vi "subGetItemInfosFromProjectRef.vi"(9 "All Files in Dir":path[](array[path]), 10 "Source dist":map{string, set{string}}(c390), 11 "TargetFile info in":T1) -> (1 "Project refs":refnum<vi>[](array[refnum]), 2 "Local Host App Instance":refnum<vi>, 3 "TargetFile info":T1)   [LabVIEW 2020, in "SolutionBuilder.lvlib"]
uses:
  SolutionBuilder.lvlib
  ItemInfo.ctl
  ProjectInfo.ctl
  FileInfo.ctl
  <vilib>/Utility/miscctls.llb/LVMapReplaceAction.ctl
  2df07852-fbbc-4590-81e1-2119d6acaec0.vi
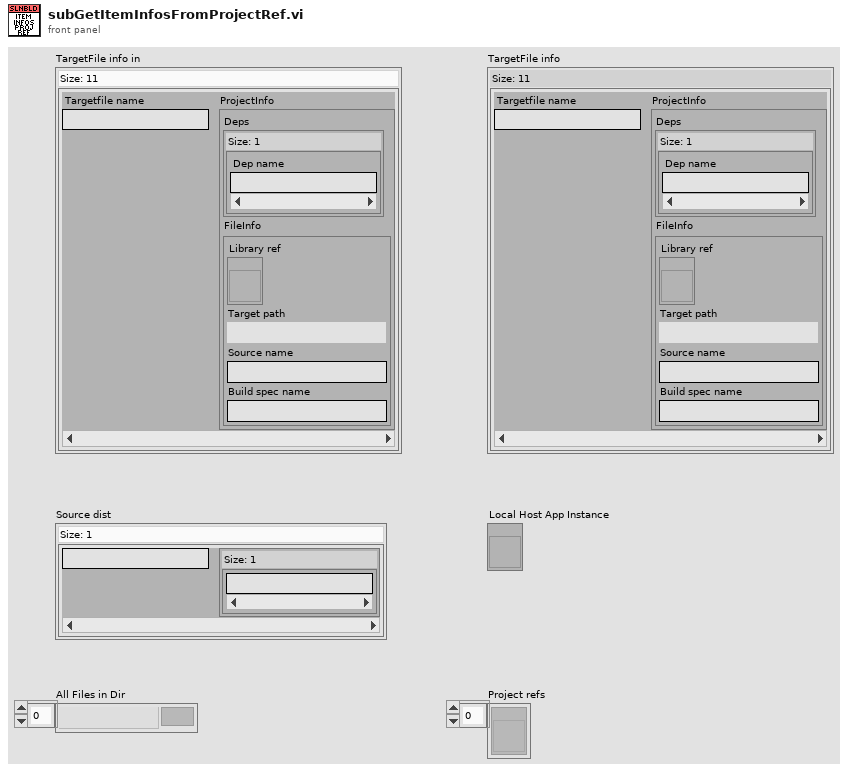
[diagram p1: front panel]
types:
  T1 = typedef "SolutionBuilder.lvlib/ItemInfo.ctl" = map{string, T2}
  T2 = typedef "SolutionBuilder.lvlib/ProjectInfo.ctl" = cluster{"Deps":set{string}, "FileInfo":T3}
  T3 = typedef "SolutionBuilder.lvlib/FileInfo.ctl" = cluster{"Library ref":refnum<vi>, "Target path":path, "Source name":string, "Build spec name":string}
  T4 = typedef "LVMapReplaceAction.ctl" = enum32{"Modify Entry only if found", "Add or Modify Entry", "Delete Entry"}
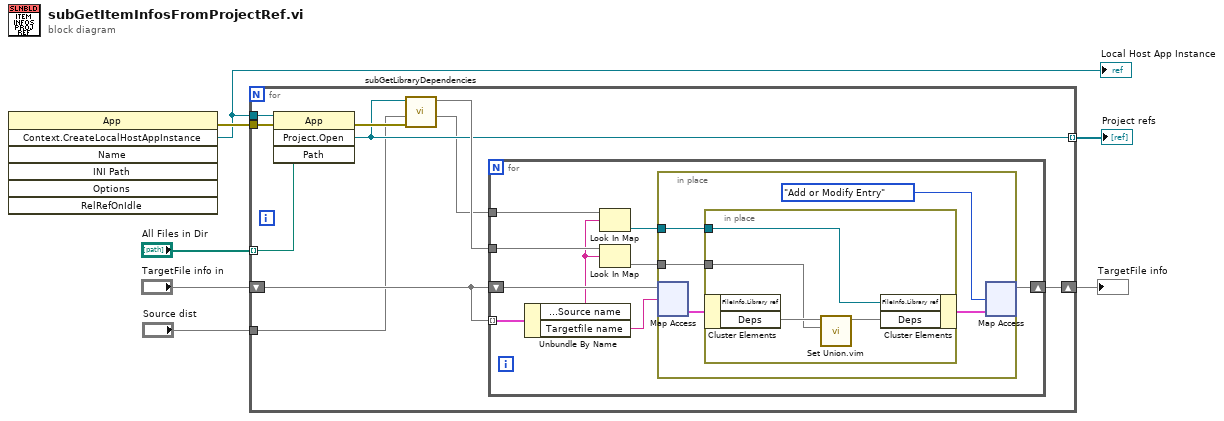
[diagram p0: block diagram]
diagram:
  n1 = invoke class="App" method="Context.CreateLocalHostAppInstance"() -> (error out=w6:errorcluster, "Create Context"=w5:refnum<vi>)  [unwired: 7 in, 5 out]
  "Local Host App Instance" <- w5
  n2 = for {
    tunnel: "All Files in Dir" -> [w17] mode=indexing
    tunnel: w6 -> [w16]
    tunnel: w5 -> [w15]
    shift-right: [w13] -> w4
    shift-left: "TargetFile info in" -> [w11]
    tunnel: [w10] -> w2 mode=indexing
    tunnel: "Source dist" -> [w8]
    n3 = invoke class="App" method="Project.Open"(reference=w15, error in=w16, "Path"=w17) -> (error out=w14:errorcluster, "Project:Open"=w10:refnum<vi>)  [unwired: 1 in, 2 out]
    n4 = call "subGetLibraryDependencies.vi"("error in (no error)"=w14, "Source dist"=w8, "Project ref"=w10) -> ("Library refs"=w9:map{string, refnum<vi>}, "Deps"=w12:map{string, set{string}})  [unwired: 6 in, 1 out]
    n5 = for {
      tunnel: w12 -> [w23]
      shift-right: [w24] -> w13
      shift-left: w11 -> [w26]
      tunnel: w11 -> [w21] mode=indexing
      tunnel: w9 -> [w20]
      n6 = Unbundle By Name(w21) -> ("ProjectInfo.FileInfo.Source name"=w19:string, "Targetfile name"=w25:string)
      n7 = Look In Map(map=w20, key=w19) -> (value=w18:refnum<vi>)  [unwired: 1 in, 1 out]
      n8 = Look In Map(map=w23, key=w19) -> (value=w22:set{string})  [unwired: 1 in, 1 out]
      n9 = in-place {
        in-place-border: w22 -> [w30]
        in-place-border: w18 -> [w27]
        n10 = in-place-map #1(w26, w25) -> (w31:T2)  [unwired: 1 in, 1 out]
        n11 = in-place {
          in-place-border: w30 -> [w34]
          in-place-border: w27 -> [w32]
          n12 = in-place-cluster #2(w31) -> ("Deps"=w35:set{string})  [unwired: 1 out]
          n13 = call "Set Union.vim"("set 2"=w34, "set 1"=w35) -> ("union"=w33:set{string})  [unwired: 9 in]
          n14 = in-place-cluster #2("FileInfo.Library ref"=w32, "Deps"=w33) -> (w29:T2)
        }
        n15 = in-place-map #1(w29, LVMapReplaceAction."Add or Modify Entry" ("action")) -> (w24:T1)  [unwired: 2 out]
      }
    }
  }
  "TargetFile info" <- w4
  "Project refs" <- w2
